vi "emp.vi"(7 "LabVIEW Web Service Request":refnum<class "Web Request.lvclass">) -> (1 "output":string, 2 "Slide":dbl)   [LabVIEW 2018]
uses:
  <vilib>/wsapi/Web Request.lvclass
  Globals.vi
panel:
  # "Each additional control wired to the connector pane will be available as an input in the URL. To include an indicator in terminal-mode output (the default setting), it must also be wired to the connector pane."
  # "Use the Web Service Request input terminal to call the VIs on the Web Services palette. Do not remove it from the connector pane unless you don't need access to the palette."
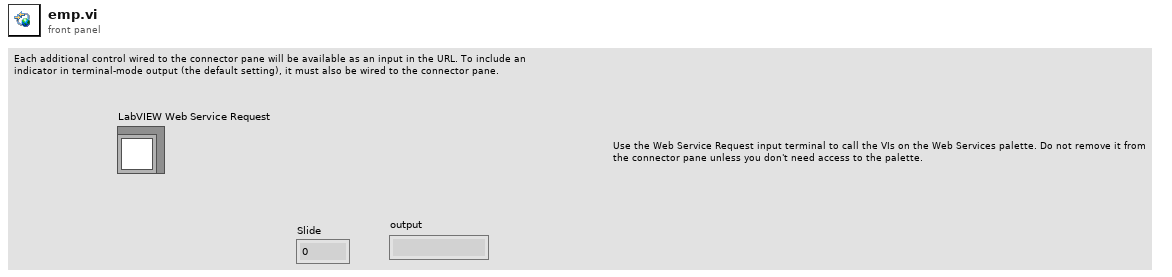
[diagram p1: front panel]
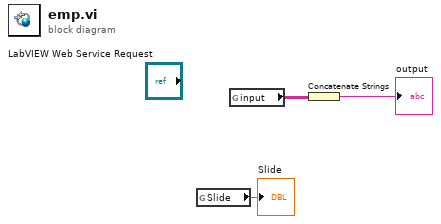
[diagram p0: block diagram]
diagram:
  n1 = global read "Globals.vi" "Slide"() -> (→"Slide":dbl)
  n2 = global read "Globals.vi" "input"() -> (w2:string[][])
  n3 = Concatenate Strings(w2) -> (→"output":string)
